vi "Get Restore Point.vi"(8 "error in (no error)":errorcluster, 9 "Active Unique ID":string, 11 "Test Executive in":refnum<class "Test Executive.lvclass">) -> (0 "error out":errorcluster, 1 "Active Unique ID out":string, 2 "Test":refnum<class "Executioner.lvclass">, 3 "Test Executive out":refnum<class "Test Executive.lvclass">, 4 "Restore Point":bool, 6 "Complete":bool)   [LabVIEW 2017, in "Test Executive.lvlib" / "Test Executive.lvclass"]
uses:
  <vilib>/gpm_packages/@cs/test-executive/Source/Test Executive/TestExecutive/Test Executive.lvclass
  <vilib>/gpm_packages/@cs/test-executive/Source/Test Executive/Executioner/Executioner.lvclass
  <vilib>/gpm_packages/@cs/test-executive/Source/Test Executive/TestExecutive/Test Executive.lvclass/Test Executive.ctl
  <vilib>/gpm_packages/@cs/linked-list/Source/Linked List/Linked List Ref/Linked List Ref.lvclass
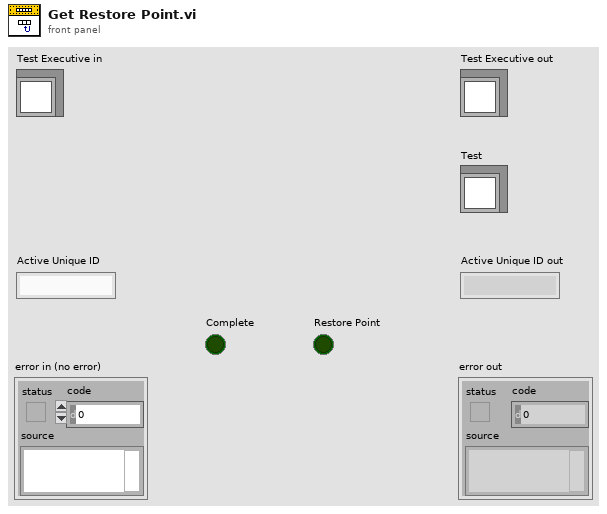
[diagram p1: front panel]
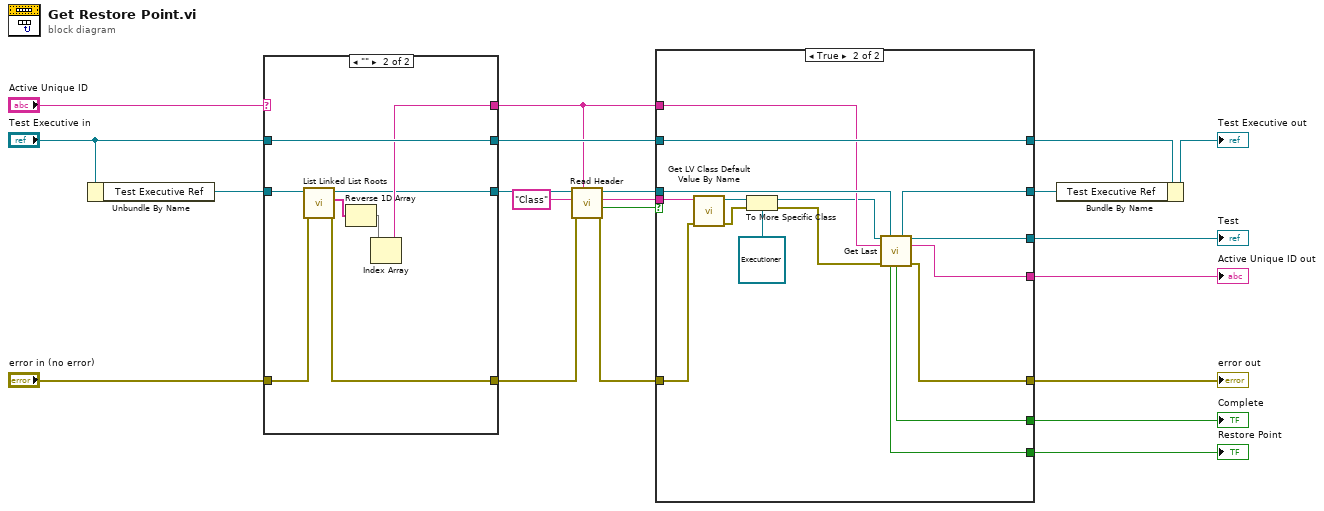
[diagram p0: block diagram]
diagram:
  n1 = Unbundle By Name("Test Executive in") -> ("Test Executive Ref"=w20:refnum<data-value>)
  n2 = case shown="\"\"" "Active Unique ID" {
    selector: "Active Unique ID" -> [w24 _]
    tunnel: "Test Executive in" -> [w25 w33]
    tunnel: w20 -> [w23 w32]
    tunnel: [w25 w33] -> w10
    tunnel: "error in (no error)" -> [w22 w31]
    tunnel: [w24 w29] -> w5
    tunnel: [w23 w28] -> w17
    tunnel: [w22 w27] -> w13
    frame Default {
    }
    frame "" {
      n3 = call <vilib>:"List Linked List Roots.vi"("error in (no error)"=w31, "Linked List Ref"=w32) -> ("error out"=w27:errorcluster, "Root IDs"=w30:string[], "Linked List Ref out"=w28:refnum<data-value>)  [unwired: 6 in, 1 out]
      n4 = Reverse 1D Array(array=w30) -> (reversed array=w26:string[])
      n5 = Index Array(array=w26) -> (element=w29:string)  [unwired: 1 in]
    }
  }
  n6 = call <vilib>:"Read Header.vi"("Linked List ID"=w5, "error in (no error)"=w13, "Header Name"="Class", "Linked List Ref"=w17) -> ("error out"=w14:errorcluster, "found"=w15:bool, "Header Value"=w11:string, "Linked List Ref out"=w12:refnum<data-value>)  [unwired: 4 in]
  n7 = case shown="True" w15 {
    tunnel: w14 -> [w35 w49]
    tunnel: w12 -> [w36 w47]
    tunnel: w11 -> [_ w52]
    tunnel: w10 -> [w37 w53]
    tunnel: [w37 w53] -> w7
    tunnel: [w36 w46] -> w9
    tunnel: [w35 w43] -> w6
    tunnel: w5 -> [w34 w44]
    tunnel: [_ w42] -> w4
    tunnel: [w34 w41] -> w3
    tunnel: [_ w40] -> w2
    tunnel: [_ w39] -> w1
    frame False {
    }
    frame True {
      n8 = call <vilib>:"Get LV Class Default Value By Name.vi"("error in (no error)"=w49, "class name"=w52) -> ("error out"=w48:errorcluster, "object"=w51:refnum<class>)  [unwired: 8 in]
      n9 = To More Specific Class(target class=refnum<class "Executioner.lvclass"> refnum ("Test Executive.lvlib:Executioner.lvclass"), reference=w51, error in=w48) -> (specific class reference=w38:refnum<class "Executioner.lvclass">, error out=w45:errorcluster)
      n10 = call-dynamic "Get Last.vi"("Executioner in"=w38, "Linked List Ref"=w47, "Active Unique ID"=w44, "error in (no error)"=w45) -> ("Linked List Ref out"=w46:refnum<data-value>, "Executioner out"=w42:refnum<class "Executioner.lvclass">, "Active Unique ID out"=w41:string, "Restore Point"=w40:bool, "Complete"=w39:bool, "error out"=w43:errorcluster)  [unwired: 4 in, 2 out]
    }
  }
  "error out" <- w6
  "Active Unique ID out" <- w3
  "Test" <- w4
  "Restore Point" <- w2
  "Complete" <- w1
  n11 = Bundle By Name(cluster=w7, "Test Executive Ref"=w9) -> (→"Test Executive out":refnum<class "Test Executive.lvclass">)
